vi "ConfigureTraceType.vi"(8 "error in (no error)":errorcluster, 11 "Keysight44xx in":refnum<class "Keysight44xx.lvclass">) -> (0 "error out":errorcluster, 3 "Keysight44xx out":refnum<class "Keysight44xx.lvclass">)   [LabVIEW 2018, in "SpecAnPlugins.lvlib" / "Keysight44xx.lvclass"]
doc: "This function configures the Trace Type attribute such as Video Average, Minimum Hold, Clear Write, etc."
uses:
  Keysight44xx.lvclass
  C:/Users/ico/Documents/Projects/NistPluggableModules/SpecAn/SpecAnPlugins/SpecAnBaseClass/SpecAnBase.lvclass
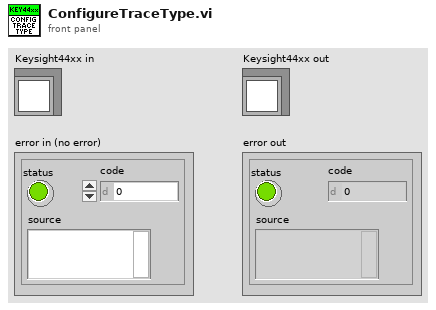
[diagram p1: front panel]
types:
  T1 = typedef "SpecAnPlugins.lvlib/SpecAnBase.lvclass/Acquisition.ctl" = cluster{"Handle":string, "Connected":bool, "Enabled":bool, "SweepModeContinuous":bool, "NumberOfSweeps":i32, "DetectorTypeAuto":bool, "DetectorType":i32, "VerticalScale":i32, "MaximumTime(seconds)":dbl}
  T2 = typedef "SpecAnPlugins.lvlib/SpecAnBase.lvclass/Trace.ctl" = cluster{"TraceName":string, "TraceSize":i32, "TraceType":i32}[]
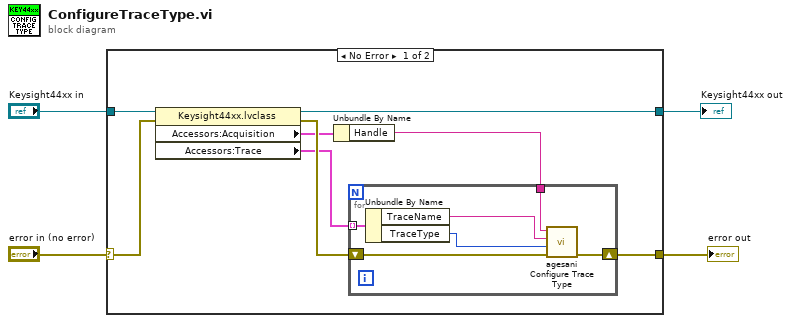
[diagram p0: block diagram]
diagram:
  n1 = case shown="No Error" "error in (no error)" {
    selector: "error in (no error)" -> [w11 w19]
    tunnel: "Keysight44xx in" -> [w12 w20]
    tunnel: [w9 w19] -> w2
    tunnel: [w10 w20] -> w1
    frame No Error {
      n2 = property class="Keysight44xx.lvclass"(reference=w12, error in=w11) -> (reference out=w10:refnum<class "Keysight44xx.lvclass">, error out=w8:errorcluster, "Accessors:Acquisition"=w7:T1, "Accessors:Trace"=w6:T2)
      n3 = Unbundle By Name(w7) -> ("Handle"=w5:string)
      n4 = for {
        shift-right: [w18] -> w9
        shift-left: w8 -> [w17]
        tunnel: w6 -> [w16] mode=indexing
        tunnel: w5 -> [w15]
        n5 = Unbundle By Name(w16) -> ("TraceName"=w14:string, "TraceType"=w13:i32)
        n6 = call <instrlib>:"agesani Configure Trace Type.vi"("error in (no error)"=w17, "trace type (Clear Write)"=w13, "trace name (\"\")"=w14, "instrument handle"=w15) -> ("error out"=w18:errorcluster)  [unwired: 7 out]
      }
    }
    frame Error {
    }
  }
  "error out" <- w2
  "Keysight44xx out" <- w1
